vi "pmu_Configuration Block.vi"(9 "CFG class":T1={"station name"="", "PMU ID"=0, "time base"=10000000, "nominal frequency"=enum."60 Hz", "reporting rate"=60, "phasor number"=0, "analog number"=0, "digital number"=0, "channel names"=[], "phasor units"=[], "analog units"=[], "digital units"=[], "data format"=15, "number of PMUs"=1} {"digital units" format="%.0x"; "analog units" format="%.0x"; "phasor units" format="%.0x"}, 10 "configuration change count":u16) -> (2 "data":u8[](array[numeric]))   [LabVIEW 2011, in "NI_EP_PMU.lvlib"]
doc: "This VI builds IEEE C37.118-2005 configuration message frame sent by the PMU."
uses:
  <vilib>/addons/Electrical Power/PMU/NI_EP_PMU.lvlib
  <vilib>/addons/Electrical Power/PMU/Common/Controls/pmu_CFG Class.ctl
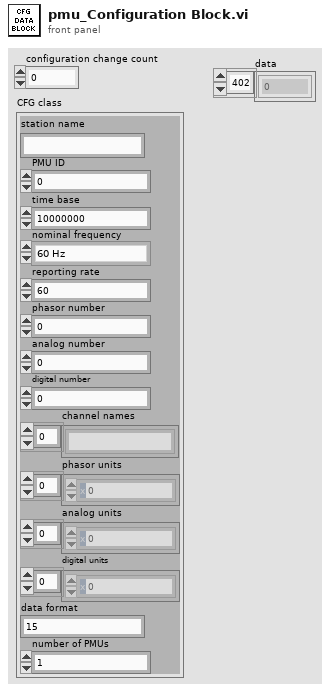
[diagram p1: front panel]
types:
  T1 = typedef "NI_EP_PMU.lvlib/pmu_CFG Class.ctl" = cluster{"station name":string, "PMU ID":u16, "time base":u32, "nominal frequency":enum16{"50 Hz", "60 Hz"}, "reporting rate":i16, "phasor number":u16, "analog number":u16, "digital number":u16, "channel names":string[], "phasor units":u32[], "analog units":u32[], "digital units":u32[], "data format":u16, "number of PMUs":u16}
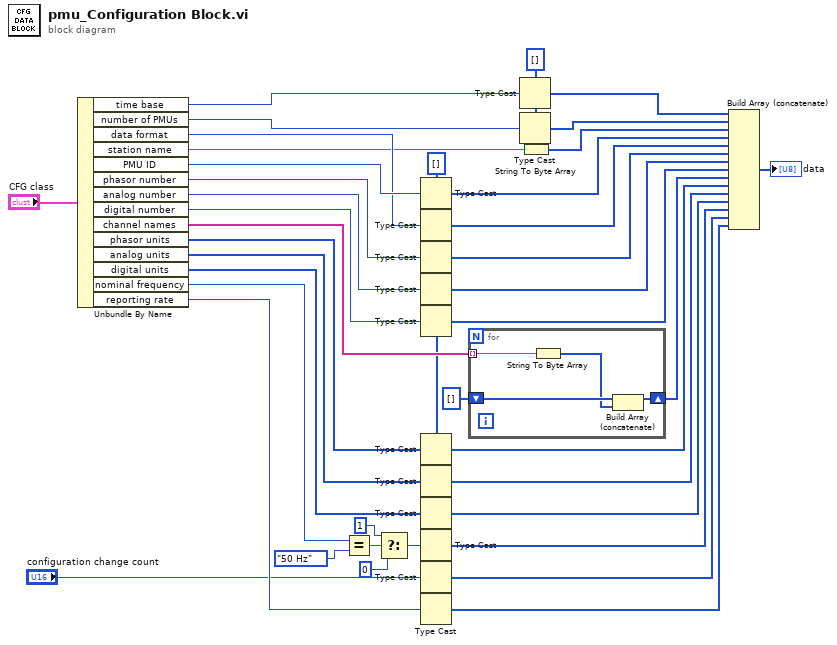
[diagram p0: block diagram]
diagram:
  w25 = u8[] [] ("appended array")
  w37 = u8[] [] ("appended array")
  n1 = Unbundle By Name("CFG class") -> ("time base"=w12:u32, "number of PMUs"=w11:u16, "data format"=w10:u16, "station name"=w9:string, "PMU ID"=w24:u16, "phasor number"=w21:u16, "analog number"=w19:u16, "digital number"=w17:u16, "channel names"=w39:string[], "phasor units"=w34:u32[], "analog units"=w32:u32[], "digital units"=w30:u32[], "nominal frequency"=w7:enum16{"50 Hz", "60 Hz"}, "reporting rate"=w15:i16)
  n2 = Equal?(x=w7, y=enum16{"50 Hz", "60 Hz"}."50 Hz" ("nominal frequency")) -> (x = y?=w6:bool)
  n3 = Select(t=u16 1, s=w6, f=u16 0) -> (s? t:f=w2:u16)
  n4 = Type Cast(type=w25, x=w24) -> (*(type *) &x=w23:u8[])
  n5 = Type Cast(type=w25, x=w10) -> (*(type *) &x=w22:u8[])
  n6 = Type Cast(type=w25, x=w21) -> (*(type *) &x=w20:u8[])
  n7 = Type Cast(type=w25, x=w19) -> (*(type *) &x=w18:u8[])
  n8 = Type Cast(type=w25, x=w17) -> (*(type *) &x=w16:u8[])
  n9 = Type Cast(type=w25, x=w34) -> (*(type *) &x=w33:u8[])
  n10 = Type Cast(type=w25, x=w32) -> (*(type *) &x=w31:u8[])
  n11 = Type Cast(type=w25, x=w30) -> (*(type *) &x=w29:u8[])
  n12 = Type Cast(type=w25, x=w2) -> (*(type *) &x=w28:u8[])
  n13 = Type Cast(type=w25, x="configuration change count") -> (*(type *) &x=w27:u8[])
  n14 = Type Cast(type=w25, x=w15) -> (*(type *) &x=w26:u8[])
  n15 = for {
    shift-right: [w43] -> w40
    shift-left: u8[] [] -> [w44]
    tunnel: w39 -> [w42] mode=indexing
    n16 = String To Byte Array(string=w42) -> (unsigned byte array=w41:u8[])
    n17 = Build Array (concatenate)(w44, w41) -> (w43:u8[])
  }
  n18 = Type Cast(type=w37, x=w12) -> (*(type *) &x=w35:u8[])
  n19 = Type Cast(type=w37, x=w11) -> (*(type *) &x=w36:u8[])
  n20 = String To Byte Array(string=w9) -> (unsigned byte array=w8:u8[])
  n21 = Build Array (concatenate)(w35, w36, w8, w23, w22, w20, w18, w16, w40, w33, w31, w29, w28, w27, w26) -> (→"data":u8[])
